vi "Obtain Msg Queue DVR.vi"(10 "Msg Queue DVR Alias":string) -> (0 "error out":errorcluster, 2 "Msg Queue DVR":refnum<data-value>)   [LabVIEW 2021, in "jettl.lvlib"]
uses:
  jettl.lvlib
  Actor/Msg/Msg.lvclass
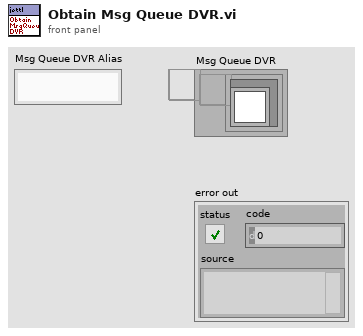
[diagram p1: front panel]
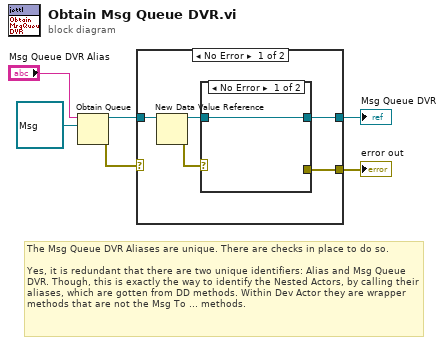
[diagram p0: block diagram]
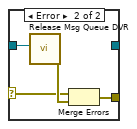
[diagram p2: hidden frame]
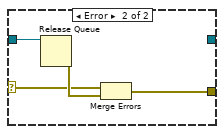
[diagram p3: hidden frame]
diagram:
  # "The Msg Queue DVR Aliases are unique. There are checks in place to do so.\n\nYes, it is redundant that there are two unique identifiers: Alias and Msg Queue DVR. Though, this is exactly the way to identify the Nested Actors, by calling their aliases, which are gotten from DD methods. Within Dev Actor they are wrapper methods that are not the Msg To ... methods."
  n1 = Obtain Queue(name (unnamed)="Msg Queue DVR Alias", element data type=refnum<class "Msg.lvclass"> refnum ("Artifex Actor Model.lvlib:Msg.lvclass")) -> (queue out=w4:refnum<queue>, error out=w6:errorcluster)  [unwired: 3 in, 1 out]
  n2 = case shown="No Error" w6 {
    selector: w6 -> [_ w17]
    tunnel: w4 -> [w11 w20]
    tunnel: [w8 _] -> w3
    tunnel: [w9 w19] -> w2
    frame No Error {
      n3 = New Data Value Reference(data value=w11) -> (data value reference=w7:refnum<data-value>, error out=w10:errorcluster)  [unwired: 1 in]
      n4 = case shown="No Error" w10 {
        selector: w10 -> [_ w13]
        tunnel: [_ w15] -> w9
        tunnel: [w12 _] -> w8
        tunnel: w7 -> [w12 w16]
        frame No Error {
        }
        frame Error {
          n5 = call "Release Msg Queue DVR.vi"("Msg Queue DVR"=w16) -> ("error out"=w14:errorcluster)  [unwired: 10 in]
          n6 = Merge Errors(w13, w14) -> (w15:errorcluster)
        }
      }
    }
    frame Error {
      n7 = Release Queue(queue=w20) -> (error out=w18:errorcluster)  [unwired: 2 in, 2 out]
      n8 = Merge Errors(w17, w18) -> (w19:errorcluster)
    }
  }
  "Msg Queue DVR" <- w3
  "error out" <- w2
